vi "FGV_CI Encoder position.vi"(7 "Function":T1, 8 "error in":errorcluster) -> (0 "error out":errorcluster, 2 "Acquired Data":dbl[](array[numeric]))   [LabVIEW 2017]
doc: "This example demonstrates how to use a counter input along with an external clock to continually sample the angular position measured from an encoder.\n\nFor instructions on how to connect your signals to the DAQ device, refer to your device documentation."
uses:
  Controls/FV_CI Encoder Position.ctl
  <vilib>/DAQmx/read.llb/DAQmx Read (Counter 1D DBL 1Chan NSamp).vi
  <vilib>/DAQmx/create/channels.llb/DAQmx Create Channel (CI-Position-Linear Encoder).vi
  <vilib>/DAQmx/configure/timing.llb/DAQmx Timing (Sample Clock).vi
  <vilib>/DAQmx/miscellaneous.llb/DAQmx Fill In Error Info.vi
  <resource>/objmgr/daqmx.rc
panel:
  in  "Z Index Terminal":tag="PFI9"
  in  "Z Index Enable":bool
  in  "Pulses Per Revolution":u32=24
  in  "B Input Terminal":tag="PFI10"
  in  "A Input Terminal":tag="PFI8"
  in  "Counter":tag="Dev1/ctr0"
  in  "Trigger Type":enum32{"No Trigger", "Digital Arm Start"}(tab)
  in  "Edge":i32(ring)=10280 items=["Rising"=10280, "Falling"=10171]
  in  "Digital Trigger Source":tag
  in  "Samples per Loop":i32=100
  in  "Sample Rate":dbl=1000.0
  in  "Sample Clock Source":tag="PFI0"
  # "Channel Settings"
  # "Acquired Data"
  # "Timing Settings"
  # "Trigger Settings"
  # "To configure and use a trigger or the count reset you must have the necessary tab selected above.  Not all hardware supports the above options--refer to your device documentation for more info."
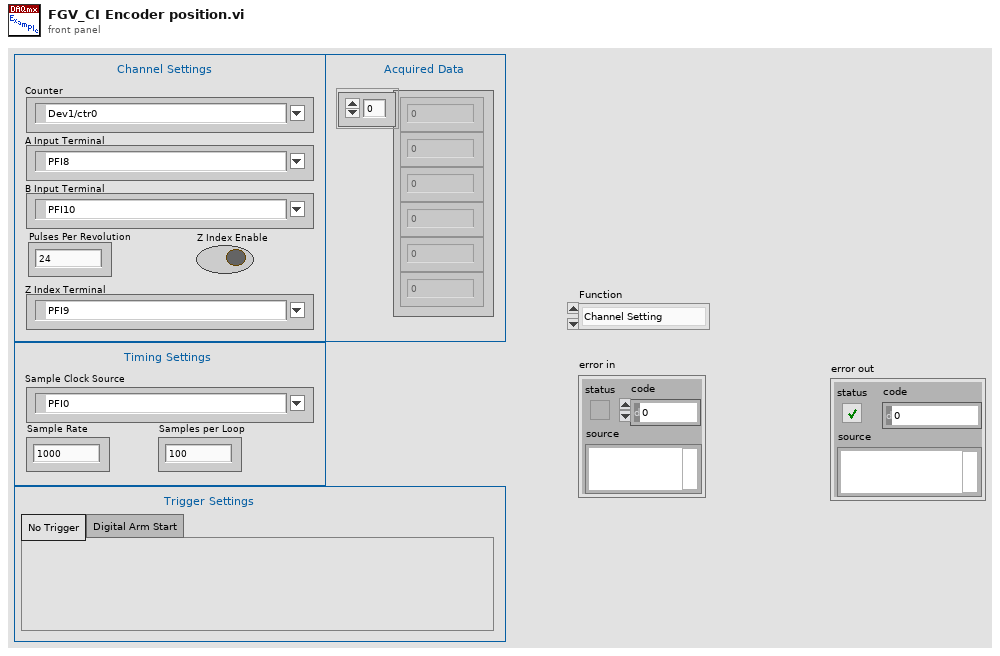
[diagram p1: front panel]
types:
  T1 = typedef "FV_CI Encoder Position.ctl" = enum16{"Channel Setting", "Timing Setting", "Trigger Setting", "Task Start", "Acquire Data", "Task Release"}
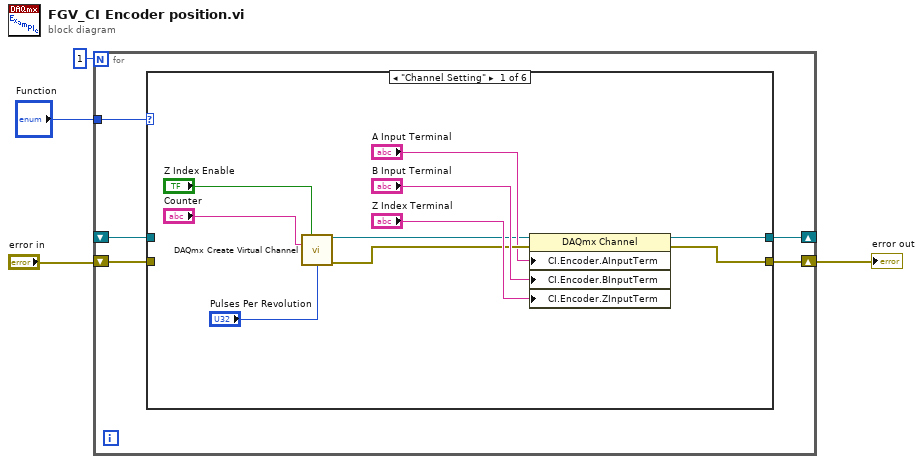
[diagram p0: block diagram]
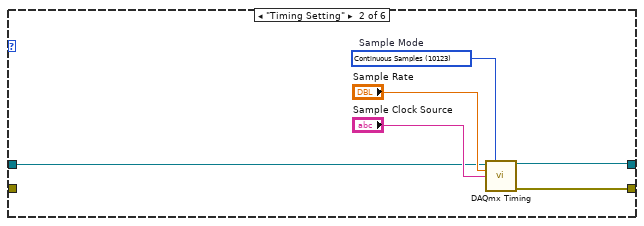
[diagram p2: hidden frame]
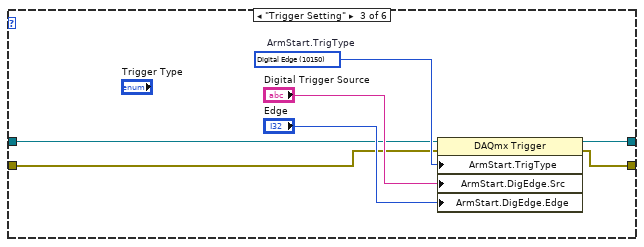
[diagram p3: hidden frame]
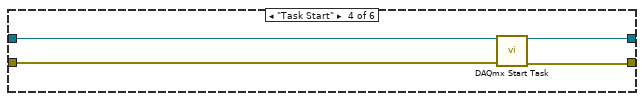
[diagram p4: hidden frame]
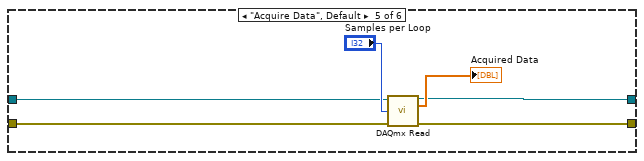
[diagram p5: hidden frame]
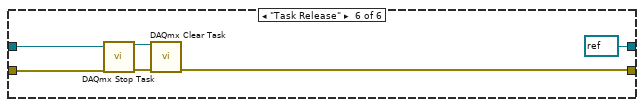
[diagram p6: hidden frame]
diagram:
  n1 = for {
    N: 1 -> [_]
    tunnel: "Function" -> [w9]
    shift-right: [w8] -> _
    shift-left: _ -> [w7]
    shift-right: [w6] -> w2
    shift-left: "error in" -> [w5]
    n2 = case shown="\"Channel Setting\"" w9 {
      tunnel: [w11 w22 w29 w36 w40 refnum<k21> refnum ("task out")] -> w8
      tunnel: w7 -> [_ w21 w27 w35 w38 w46]
      tunnel: [w10 w20 w28 w34 w39 w44] -> w6
      tunnel: w5 -> [_ _ w26 w33 w37 w45]
      frame "Channel Setting" {
        n3 = call-poly <vilib>:"DAQmx Create Virtual Channel.vi"("z index enable"="Z Index Enable", "counter"="Counter", "distance per pulse"="Pulses Per Revolution") -> ("task out"=w13:refnum<k21>, "error out"=w15:errorcluster)  [unwired: 11 in]
        n4 = property class="DAQmx Channel"(reference=w13, error in=w15, "CI.Encoder.AInputTerm"="A Input Terminal", "CI.Encoder.BInputTerm"="B Input Terminal", "CI.Encoder.ZInputTerm"="Z Index Terminal") -> (reference out=w11:refnum<k21>, error out=w10:errorcluster)
      }
      frame "Timing Setting" {
        w23 = 10123 items=["Finite Samples"=10178, "Continuous Samples"=10123, "Hardware Timed Single Point"=12522]  # Sample Mode
        n5 = call-poly <vilib>:"DAQmx Timing.vi"("task/channels in"=w21, "sample mode"=w23, "rate"="Sample Rate", "source"="Sample Clock Source") -> ("task out"=w22:refnum<k21>, "error out"=w20:errorcluster)  [unwired: 10 in]
      }
      frame "Trigger Setting" {
        w30 = 10150 items=["Digital Edge"=10150, "None"=10230]  # ArmStart.TrigType
        n6 = property class="DAQmx Trigger"(reference=w27, error in=w26, "ArmStart.TrigType"=w30, "ArmStart.DigEdge.Src"="Digital Trigger Source", "ArmStart.DigEdge.Edge"="Edge") -> (reference out=w29:refnum<k21>, error out=w28:errorcluster)
      }
      frame "Task Start" {
        n7 = call <vilib>:"DAQmx Start Task.vi"("task/channels in"=w35, "error in"=w33) -> ("task out"=w36:refnum<k21>, "error out"=w34:errorcluster)  [unwired: 12 in]
      }
      frame "Acquire Data", Default {
        n8 = call-poly <vilib>:"DAQmx Read.vi"("task/channels in"=w38, "number of samples per channel"="Samples per Loop", "error in"=w37) -> ("task out"=w40:refnum<k21>, "data"=→"Acquired Data":dbl[], "error out"=w39:errorcluster)  [unwired: 10 in]
      }
      frame "Task Release" {
        n9 = call <vilib>:"DAQmx Stop Task.vi"("task/channels in"=w46, "error in"=w45) -> ("task out"=w48:refnum<k21>, "error out"=w47:errorcluster)  [unwired: 12 in]
        n10 = call <vilib>:"DAQmx Clear Task.vi"("task in"=w48, "error in"=w47) -> ("error out"=w44:errorcluster)  [unwired: 13 in]
      }
    }
  }
  "error out" <- w2
